vi "数据转化.vi"(11 "配方数据":string[][](table)) -> (3 "转化数据":variant[](array[variant]))   [LabVIEW 2013]
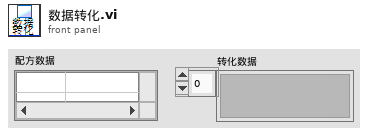
[diagram p1: front panel]
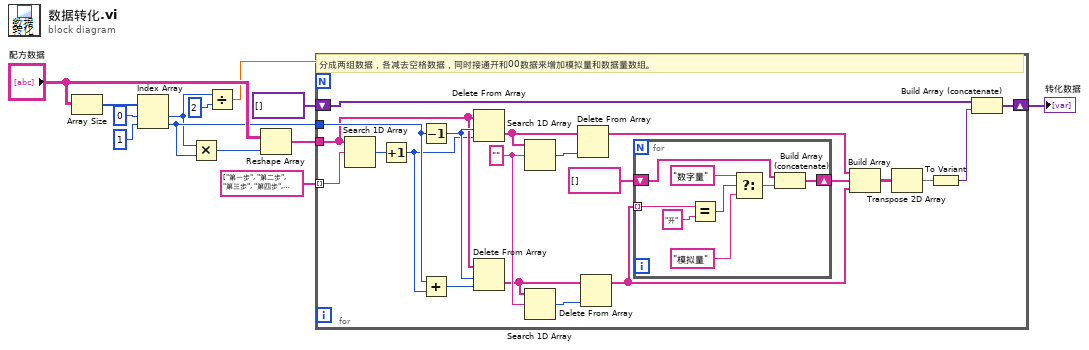
[diagram p0: block diagram]
diagram:
  n1 = Array Size(array="配方数据") -> (size(s)=w13:i32[])
  n2 = Index Array(array=w13, index #1=0 ("索引"), index #2=1 ("索引")) -> (element #1=w3:i32, element #2=w6:i32)
  n3 = Multiply(x=w3, y=w6) -> (x*y=w10:i32)
  n4 = Divide(x=w3, y=2) -> (x/y=w1:dbl)
  n5 = Reshape Array("配方数据", w10) -> (w9:string[])
  n6 = for {
    N: w1 -> [_]
    tunnel: w9 -> [w30]
    tunnel: w6 -> [w33]
    tunnel: string[] ["第一步", "第二步", "第三步", "第四步", "第五步", "第六步", "第八步", "第九步", "第十步", "第十一步", "第十二步", "第十三步", "第十四步", "第十五步", "第十六步"] -> [w29] mode=indexing
    shift-right: [w22] -> w2
    shift-left: variant[] [] -> [w20]
    w25 = ""
    # "分成两组数据，各减去空格数据，同时接通开和00数据来增加模拟量和数据量数组。"
    n7 = Search 1D Array(1D array=w30, element=w29) -> (index of element=w34:i32)  [unwired: 1 in]
    n8 = Increment(x=w34) -> (x+1=w28:i32)
    n9 = Decrement(x=w33) -> (x-1=w31:i32)
    n10 = Add(x=w33, y=w28) -> (x+y=w32:i32)
    n11 = Delete From Array(array=w30, length=w31, index=w28) -> (deleted portion=w27:string[])  [unwired: 1 out]
    n12 = Delete From Array(array=w30, length=w31, index=w32) -> (deleted portion=w24:string[])  [unwired: 1 out]
    n13 = Search 1D Array(1D array=w27, element=w25) -> (index of element=w26:i32)  [unwired: 1 in]
    n14 = Search 1D Array(1D array=w24, element=w25) -> (index of element=w19:i32)  [unwired: 1 in]
    n15 = Delete From Array(array=w27, index=w26) -> (array with subset deleted=w23:string[])  [unwired: 1 in, 1 out]
    n16 = Delete From Array(array=w24, index=w19) -> (array with subset deleted=w15:string[])  [unwired: 1 in, 1 out]
    n17 = for {
      tunnel: w15 -> [w35] mode=indexing
      shift-right: [w40] -> w16
      shift-left: string[] [] -> [w39]
      n18 = Equal?(x=w35, y="开") -> (x = y?=w42:bool)
      n19 = Select(t="数字量" ("y"), s=w42, f="模拟量") -> (s? t:f=w41:string)
      n20 = Build Array (concatenate)(w39, w41) -> (w40:string[])
    }
    n21 = Build Array(w23, w16, w15) -> (w17:string[][])
    n22 = Transpose 2D Array(2D array=w17) -> (transposed array=w14:string[][])
    n23 = To Variant(anything=w14) -> (Variant=w21:variant)
    n24 = Build Array (concatenate)(w20, w21) -> (w22:variant[])
  }
  "转化数据" <- w2
